vi "Get Server Internal UEs.vi"(11 "OOP Server in":refnum<class "HVC6.lvclass">) -> (2 "Server Internal UEs":T1, 3 "OOP Server out":refnum<class "HVC6.lvclass">)   [LabVIEW 2019, in "HVC6.lvlib" / "HVC6.lvclass"]
uses:
  HVC6.lvclass
  typeDefs/Server Internal UEs.ctl
  typeDefs/Server Internal Message.ctl
  HVC6.lvclass/HVC6.ctl
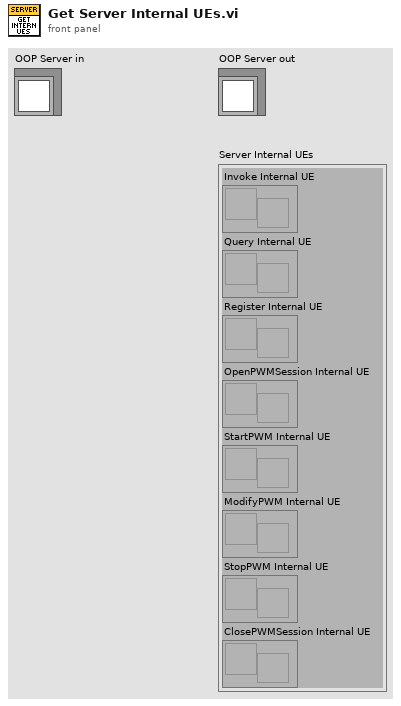
[diagram p1: front panel]
types:
  T1 = typedef "HVC6.lvlib/HVC6.lvclass/Server Internal UEs.ctl" = cluster{"Invoke Internal UE":refnum<user-event>, "Query Internal UE":refnum<user-event>, "Register Internal UE":refnum<user-event>, "OpenPWMSession Internal UE":refnum<user-event>, "StartPWM Internal UE":refnum<user-event>, "ModifyPWM Internal UE":refnum<user-event>, "StopPWM Internal UE":refnum<user-event>, "ClosePWMSession Internal UE":refnum<user-event>}
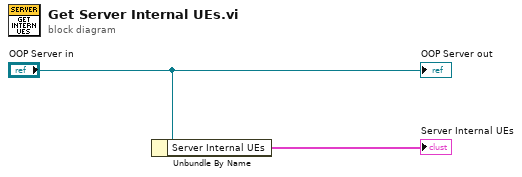
[diagram p0: block diagram]
diagram:
  n1 = Unbundle By Name("OOP Server in") -> ("Server Internal UEs"=→"Server Internal UEs":T1)
  "OOP Server out" <- "OOP Server in"
